vi "Launcher.vi"   [LabVIEW 2021]
uses:
  Main_Control/Main_Control/Main_Control.lvclass
  C:/Program Files (x86)/National Instruments/LabVIEW 2021/vi.lib/ActorFramework/Actor/Actor.lvclass
  <vilib>/ActorFramework/Actor/Actor.lvclass
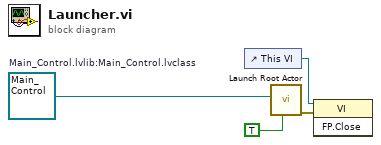
[diagram p0: block diagram]
diagram:
  w4 = refnum<class "Main_Control.lvclass"> refnum  # Main_Control.lvlib:Main_Control.lvclass
  n1 = control-ref of="This VI"() -> (w2:refnum<vi>)
  n2 = call <vilib>:"Launch Root Actor.vi"("Open Actor Core front panel? (F)"=TRUE, "Actor"=w4) -> ("error out"=w1:errorcluster)  [unwired: 8 in, 1 out]
  n3 = invoke class="VI" method="FP.Close"(reference=w2, error in=w1) -> ()  [unwired: 1 in, 3 out]
